vi "Event Handler.vi"(0 "Monkey in":refnum<class "Monkey.lvclass">, 5 "Event type":T1=enum."Message", 7 "Item Name":string, 9 "Data":variant, 11 "error in (no error)":errorcluster) -> (4 "Monkey out":refnum<class "Monkey.lvclass">, 15 "error out":errorcluster)   [LabVIEW 2020, in "Monkey.lvlib" / "Monkey.lvclass"]
doc: "This VI is the event handler of the uService: every time an event is triggered to the uService, this VI is called.\nNote: here you can access the Actor/Class data, but it will be the one coming out from Init. You cannot modify the values.\nThree different events are supported:\nI) Button Pressed: get called on a GUI button pressed. Item Name is the name (label) of the button, Data is empty.\nII) Shared Variable Updated: get called when a SV you subscribed to is updated. Item Name is the name of the SV, and Data is the value (note: you need to convert it to the proper type).\nIII) Message: get called every time a user event is generated using Send Message to Event Handler. The values of Item Name and Data are the one given to the Send Message to Event Handler.\nIV) Ready to launch?: this frame get called every time a new Run is initiated. Each uService is responsible of performing a self check before giving back the green light for the Run to start."
uses:
  Monkey.lvclass
  TALOS/TALOS_PPL.lvlibp/Father of all uServices/Father of all uServices/Event Handler Items.ctl
  Monkey Consumer Case Selector.ctl
  Run Utilities/TypeDefs/Messages/Schedule Message.ctl
  Run Utilities/TypeDefs/DAQ Control.ctl
  Run Utilities/Schedule/Schedule.lvclass
  Run Utilities/TypeDefs/Script Checker Result.ctl
  Inner stop message.ctl
  Run Utilities/Run Block/Run Block.lvclass
  TALOS/TALOS_PPL.lvlibp/Father of all uServices/Father of all uServices/Father of all uServices.lvclass
  Monkey.lvclass/Monkey.ctl
  Run Utilities/Run Utilities.lvlib
  TALOS/TALOS_PPL.lvlibp
  C:/LabVIEW Code/CIRCUS/TALOS/TALOS_PPL.lvlibp/Father of all uServices/Father of all uServices/Father of all uServices.lvclass
  C:/LabVIEW Code/CIRCUS/TALOS/TALOS_PPL.lvlibp/Ancestor/Ancestor/Ancestor.lvclass
  C:/LabVIEW Code/CIRCUS/TALOS/Actor Framework.lvlibp/1abvi3w/vi.lib/ActorFramework/Actor/Actor.lvclass
  C:/LabVIEW Code/CIRCUS/CIRCUS uServices et al/Monkey/Monkey.lvclass
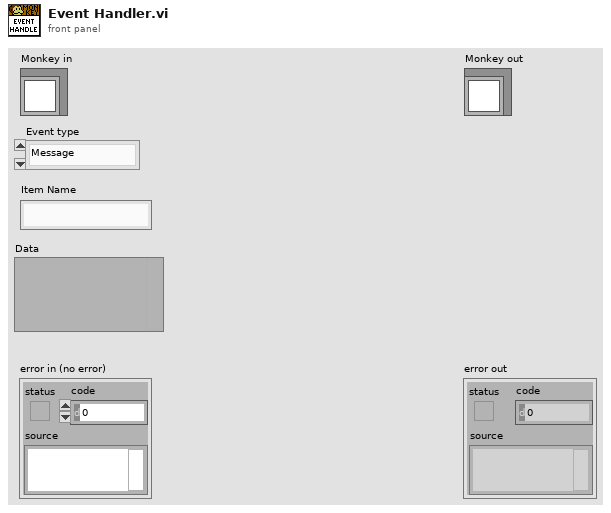
[diagram p1: front panel]
types:
  T1 = typedef "TALOS_PPL.lvlibp/Father of all uServices.lvlib/Father of all uServices.lvclass/Event Handler Items.ctl" = enum16{"Button Pressed", "Message", "Ready to launch?", "Safe Mode", "Start RUN", "Stop RUN"}
  T2 = typedef "Monkey.lvlib/Monkey.lvclass/Monkey Consumer Case Selector.ctl" = enum16{"Init", "Update GUI", "New schedule", "Check Script", "Submit Script", "Banana arrived", "Optimiser - evaluate RUN", "Optimiser - update RUN", "Quality Check", "What to do next", "Update Crit Lvl", "Skip Run", "Stop Schedule", "Skip schedule", "Append"}
  T3 = typedef "Run Utilities.lvlib/Schedule Message.ctl" = cluster{"uS Name":string, "Synchronised":bool, "DAQ Control":T4, "Schedule":refnum<class "Schedule.lvclass">, "Append to top?":bool}
  T4 = typedef "Run Utilities.lvlib/DAQ Control.ctl" = enum16{"On", "Off", "External"}
  T5 = typedef "Run Utilities.lvlib/Script Checker Result.ctl" = enum16{"Passed", "Failed", "Empty"}
  T6 = typedef "Monkey.lvlib/Monkey.lvclass/Inner stop message.ctl" = cluster{"Old value":bool, "Gracefully?":bool}
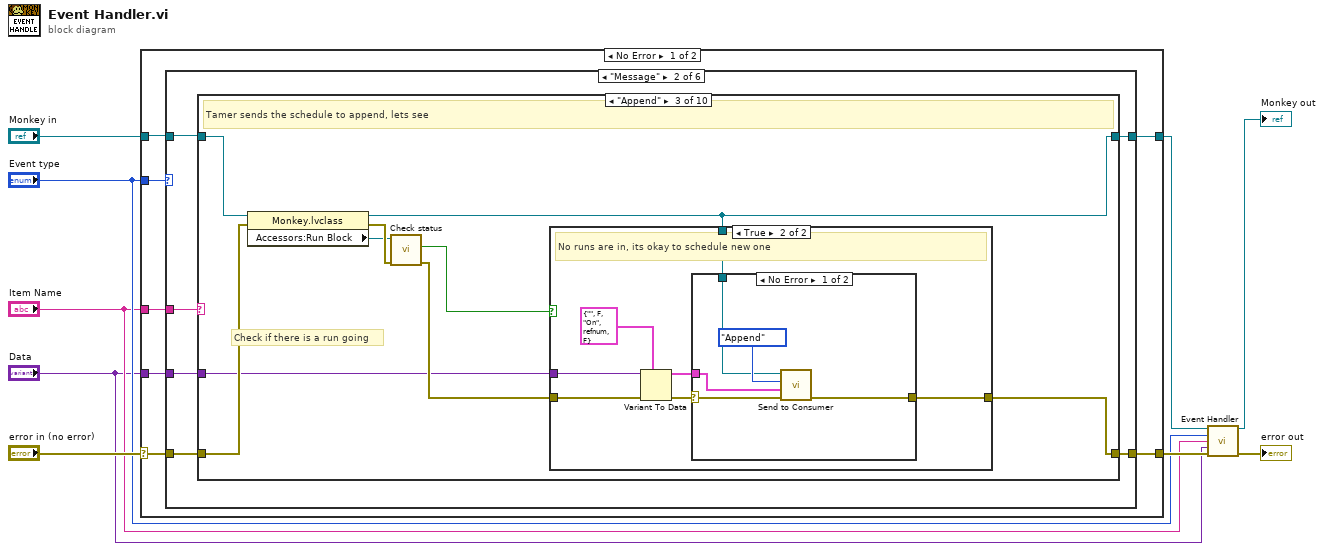
[diagram p0: block diagram]
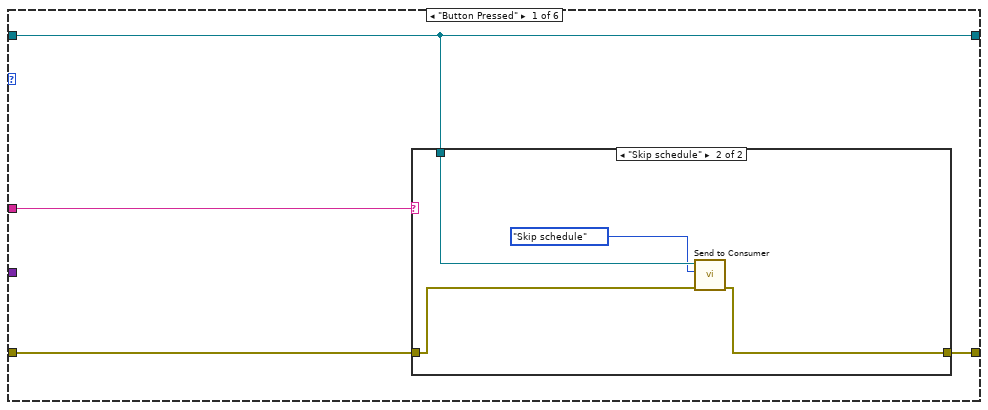
[diagram p2: hidden frame]
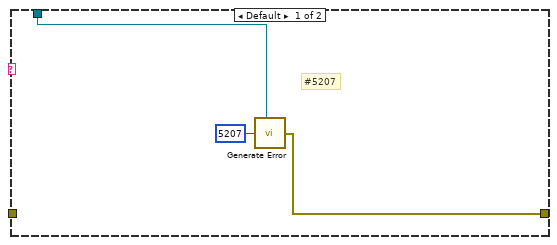
[diagram p3: hidden frame]
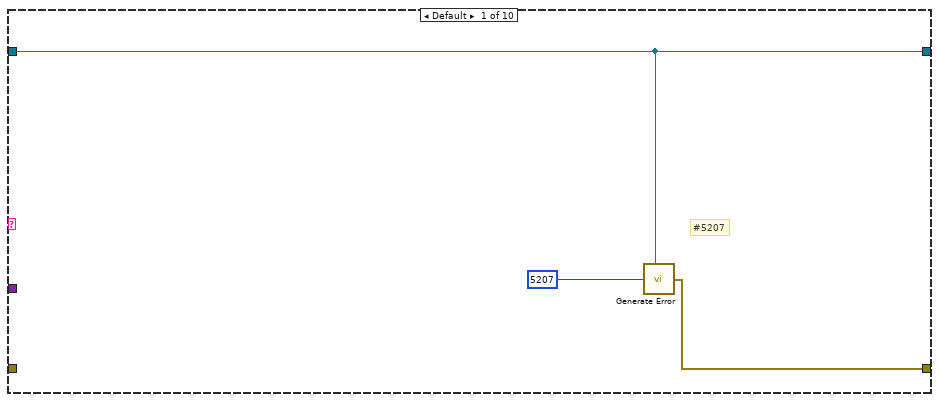
[diagram p4: hidden frame]
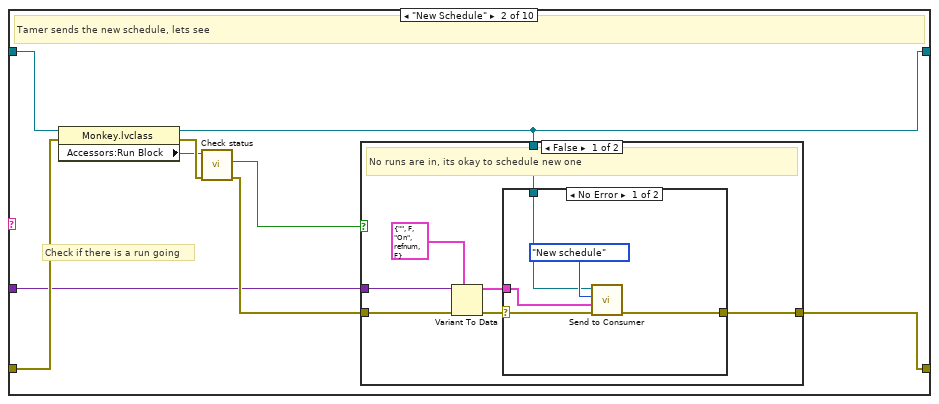
[diagram p5: hidden frame]
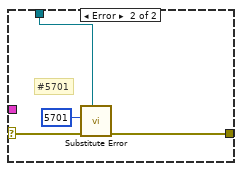
[diagram p6: hidden frame]
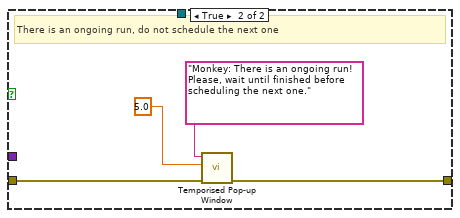
[diagram p7: hidden frame]
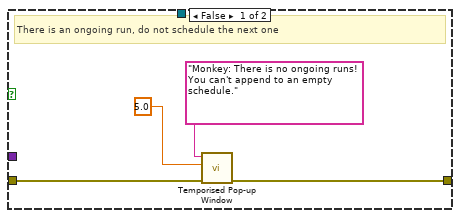
[diagram p8: hidden frame]
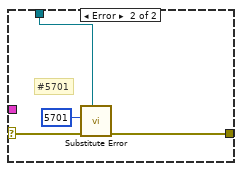
[diagram p9: hidden frame]
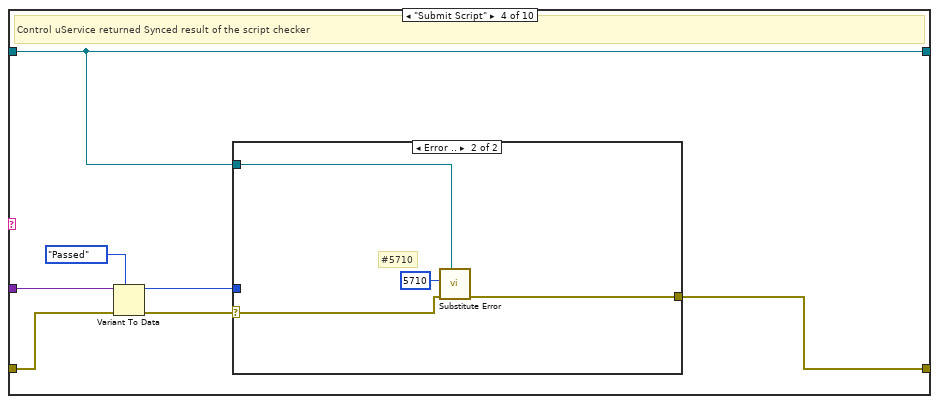
[diagram p10: hidden frame]
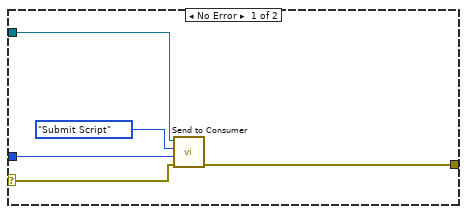
[diagram p11: hidden frame]
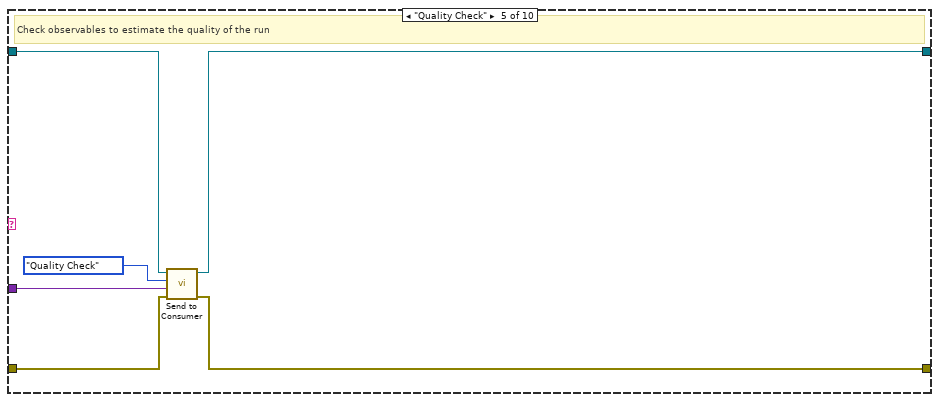
[diagram p12: hidden frame]
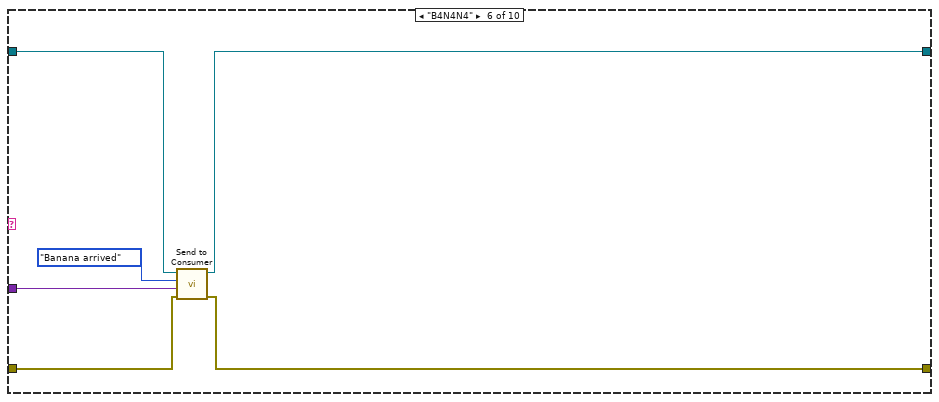
[diagram p13: hidden frame]
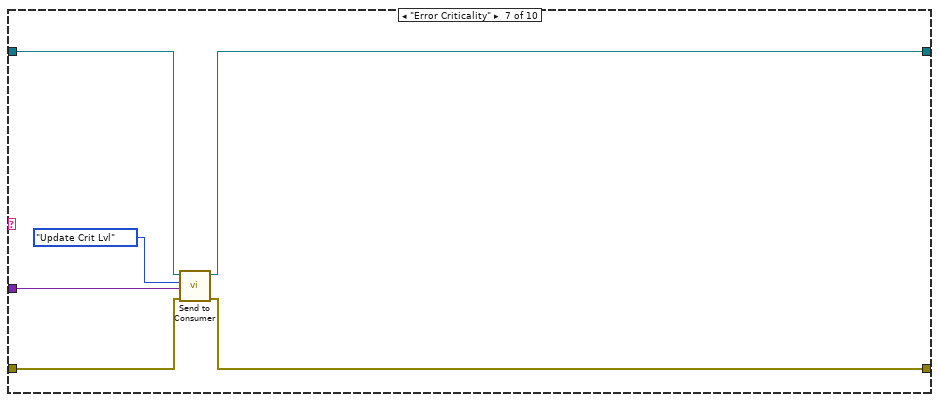
[diagram p14: hidden frame]
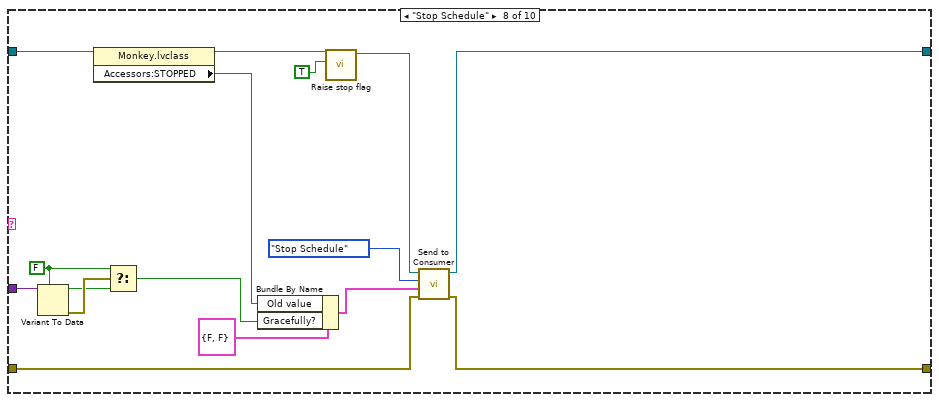
[diagram p15: hidden frame]
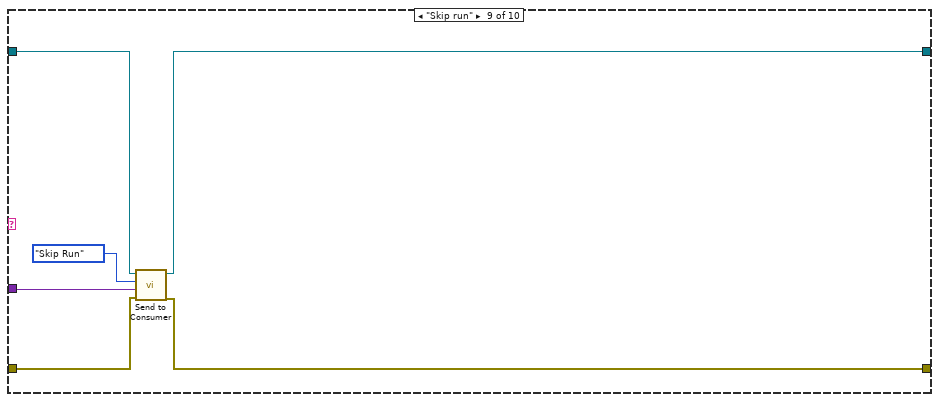
[diagram p16: hidden frame]
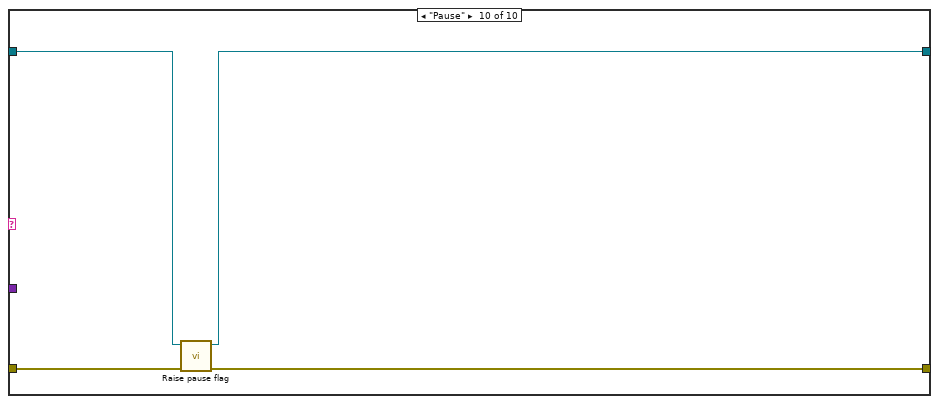
[diagram p17: hidden frame]
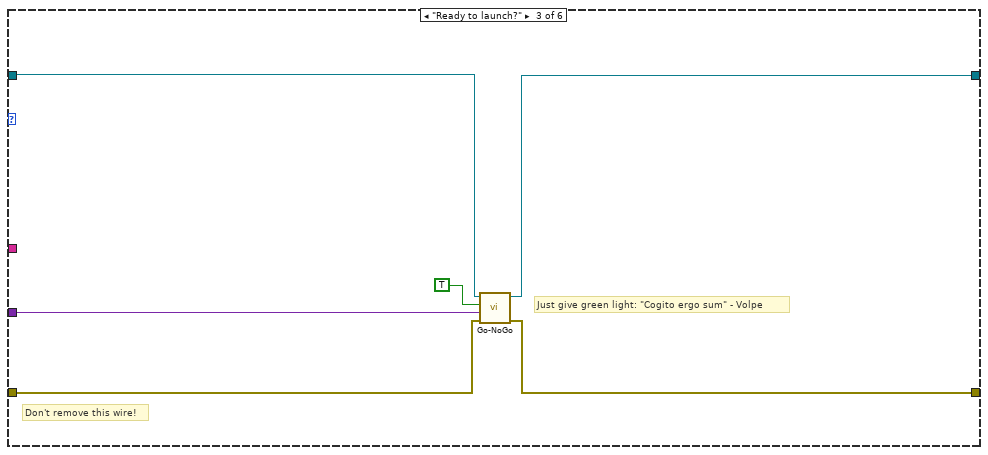
[diagram p18: hidden frame]
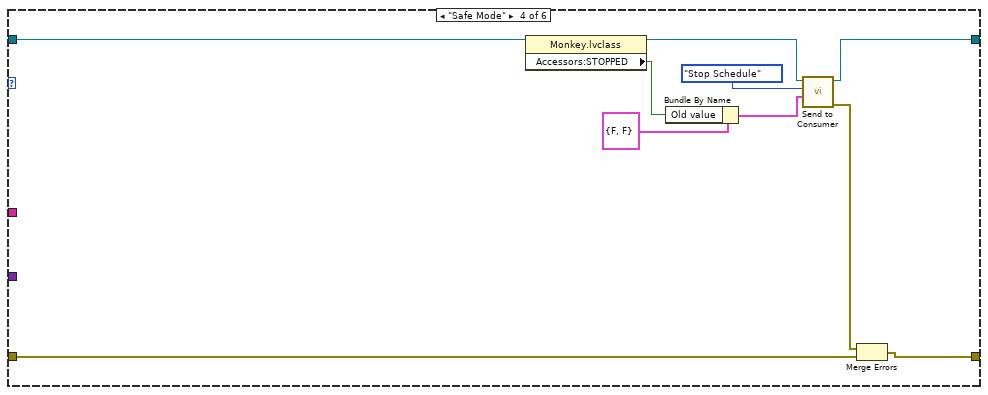
[diagram p19: hidden frame]
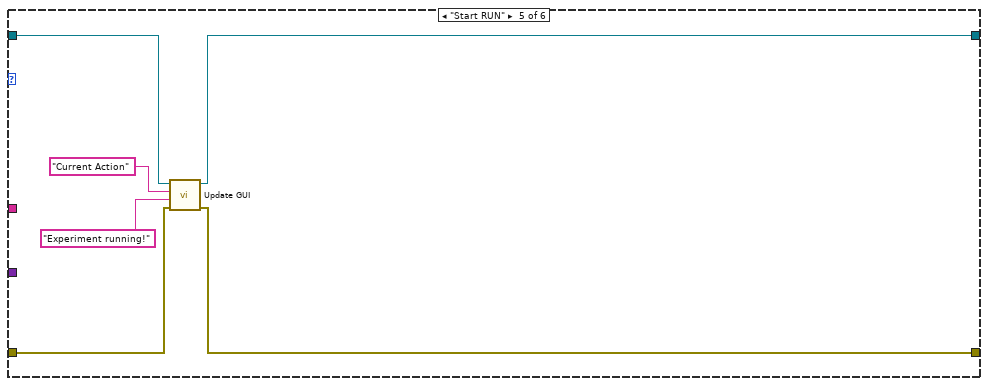
[diagram p20: hidden frame]
diagram:
  n1 = case shown="No Error" "error in (no error)" {
    selector: "error in (no error)" -> [w14 w184]
    tunnel: [w15 w184] -> w7
    tunnel: [w11 w183] -> w4
    tunnel: "Monkey in" -> [w10 w183]
    tunnel: "Event type" -> [w16 _]
    tunnel: "Item Name" -> [w13 _]
    tunnel: "Data" -> [w12 _]
    frame No Error {
      n2 = case shown="\"Message\"" w16 {
        tunnel: [w20 w29 w159 w168 w172 w179] -> w15
        tunnel: w14 -> [w18 w33 w160 w170 w175 w182]
        tunnel: w13 -> [w19 w32 _ _ _ _]
        tunnel: w10 -> [w17 w30 w158 w164 w176 w178]
        tunnel: w12 -> [_ w31 w156 _ _ _]
        tunnel: [w17 w28 w155 w166 w171 w177] -> w11
        frame "Button Pressed" {
          n3 = case shown="\"Skip schedule\"" w19 {
            tunnel: w18 -> [_ w26]
            tunnel: [w21 w25] -> w20
            tunnel: w17 -> [w22 w27]
            frame Default {
              # "#5207"
              n4 = call "Generate Error.vi"("Class"=w22, "Error Code"=5207) -> ("error out"=w21:errorcluster)  [unwired: 5 in]
            }
            frame "Skip schedule" {
              n5 = call "Send to Consumer.vi"("error in (no error)"=w26, "Case ID"=Monkey_Consumer_Case_Selector."Skip schedule" ("Monkey Consumer Case Selector"), "uService Template in"=w27) -> ("error out"=w25:errorcluster)  [unwired: 7 in, 1 out]
            }
          }
        }
        frame "Message" {
          n6 = case shown="\"Append\"" w32 {
            tunnel: w33 -> [_ w45 w74 w100 w114 w121 w128 w144 w150 w153]
            tunnel: w31 -> [_ w42 w71 w101 w116 w119 w127 w135 w149 _]
            tunnel: w30 -> [w34 w38 w67 w95 w112 w118 w124 w141 w145 w154]
            tunnel: [w35 w41 w70 w96 w113 w120 w126 w143 w148 w152] -> w29
            tunnel: [w34 w37 w66 w95 w111 w117 w123 w140 w146 w151] -> w28
            frame Default {
              # "#5207"
              n7 = call "Generate Error.vi"("Class"=w34, "Error Code"=5207) -> ("error out"=w35:errorcluster)  [unwired: 5 in]
            }
            frame "New Schedule" {
              # "Check if there is a run going"
              # "Tamer sends the new schedule, lets see"
              n8 = property class="Monkey.lvclass"(reference=w38, error in=w45) -> (reference out=w37:refnum<class "Monkey.lvclass">, error out=w43:errorcluster, "Accessors:Run Block"=w40:refnum<class "Run Block.lvclass">)
              n9 = call-dynamic "Check status.vi"("error in (no error)"=w43, "Run Block in"=w40) -> ("error out"=w44:errorcluster, "Running"=w39:bool)  [unwired: 7 in, 1 out]
              n10 = case shown="False" w39 {
                tunnel: w42 -> [w52 _]
                tunnel: [w49 w62] -> w41
                tunnel: w37 -> [w48 _]
                tunnel: w44 -> [w47 w65]
                frame False {
                  # "No runs are in, its okay to schedule new one"
                  n11 = Variant To Data(error in=w47, type=T3 {"uS Name"="", "Synchronised"=FALSE, "DAQ Control"=enum."On", "Schedule"=refnum, "Append to top?"=FALSE} ("Monkey Schedule Message"), Variant=w52) -> (data=w50:T3, error out=w51:errorcluster)
                  n12 = case shown="No Error" w51 {
                    selector: w51 -> [w55 w61]
                    tunnel: w50 -> [w54 _]
                    tunnel: w48 -> [w56 w58]
                    tunnel: [w53 w59] -> w49
                    frame No Error {
                      n13 = call "Send to Consumer.vi"("error in (no error)"=w55, "Data"=w54, "Case ID"=Monkey_Consumer_Case_Selector."New schedule" ("Monkey Consumer Case Selector"), "uService Template in"=w56) -> ("error out"=w53:errorcluster)  [unwired: 6 in, 1 out]
                    }
                    frame Error {
                      # "#5701"
                      n14 = call "Substitute Error.vi"("LabVIEW Object"=w58, "error in (no error)"=w61, "Error Code"=5701) -> ("error out"=w59:errorcluster)  [unwired: 8 in]
                    }
                  }
                }
                frame True {
                  # "There is an ongoing run, do not schedule the next one"
                  n15 = call "Temporised Pop-up Window.vi"("error in (no error)"=w65, "Timeout"=5.0, "Text"="Monkey: There is an ongoing run! Please, wait until finished before scheduling the next one.") -> ("error out"=w62:errorcluster)  [unwired: 8 in]
                }
              }
            }
            frame "Append" {
              # "Check if there is a run going"
              # "Tamer sends the schedule to append, lets see"
              n16 = property class="Monkey.lvclass"(reference=w67, error in=w74) -> (reference out=w66:refnum<class "Monkey.lvclass">, error out=w72:errorcluster, "Accessors:Run Block"=w69:refnum<class "Run Block.lvclass">)
              n17 = call-dynamic "Check status.vi"("error in (no error)"=w72, "Run Block in"=w69) -> ("error out"=w73:errorcluster, "Running"=w68:bool)  [unwired: 7 in, 1 out]
              n18 = case shown="True" w68 {
                tunnel: w71 -> [_ w85]
                tunnel: [w75 w82] -> w70
                tunnel: w66 -> [_ w81]
                tunnel: w73 -> [w78 w80]
                frame False {
                  # "There is an ongoing run, do not schedule the next one"
                  n19 = call "Temporised Pop-up Window.vi"("error in (no error)"=w78, "Timeout"=5.0, "Text"="Monkey: There is no ongoing runs! You can't append to an empty schedule.") -> ("error out"=w75:errorcluster)  [unwired: 8 in]
                }
                frame True {
                  # "No runs are in, its okay to schedule new one"
                  n20 = Variant To Data(error in=w80, type=T3 {"uS Name"="", "Synchronised"=FALSE, "DAQ Control"=enum."On", "Schedule"=refnum, "Append to top?"=FALSE} ("Monkey Schedule Message"), Variant=w85) -> (data=w83:T3, error out=w84:errorcluster)
                  n21 = case shown="No Error" w84 {
                    selector: w84 -> [w88 w94]
                    tunnel: w83 -> [w87 _]
                    tunnel: w81 -> [w89 w91]
                    tunnel: [w86 w92] -> w82
                    frame No Error {
                      n22 = call "Send to Consumer.vi"("error in (no error)"=w88, "Data"=w87, "Case ID"=Monkey_Consumer_Case_Selector."Append" ("Monkey Consumer Case Selector"), "uService Template in"=w89) -> ("error out"=w86:errorcluster)  [unwired: 6 in, 1 out]
                    }
                    frame Error {
                      # "#5701"
                      n23 = call "Substitute Error.vi"("LabVIEW Object"=w91, "error in (no error)"=w94, "Error Code"=5701) -> ("error out"=w92:errorcluster)  [unwired: 8 in]
                    }
                  }
                }
              }
            }
            frame "Submit Script" {
              # "Control uService returned Synced result of the script checker"
              n24 = Variant To Data(error in=w100, type=Script_Checker_Result."Passed" ("Script Checker Result"), Variant=w101) -> (data=w97:T5, error out=w98:errorcluster)
              n25 = case shown="Error .." w98 {
                selector: w98 -> [w103 w108]
                tunnel: w97 -> [w105 _]
                tunnel: w95 -> [w104 w109]
                tunnel: [w102 w110] -> w96
                frame No Error {
                  n26 = call "Send to Consumer.vi"("error in (no error)"=w103, "Data"=w105, "Case ID"=Monkey_Consumer_Case_Selector."Submit Script" ("Monkey Consumer Case Selector"), "uService Template in"=w104) -> ("error out"=w102:errorcluster)  [unwired: 6 in, 1 out]
                }
                frame Error {
                  # "#5710"
                  n27 = call "Substitute Error.vi"("LabVIEW Object"=w109, "error in (no error)"=w108, "Error Code"=5710) -> ("error out"=w110:errorcluster)  [unwired: 8 in]
                }
              }
            }
            frame "Quality Check" {
              # "Check observables to estimate the quality of the run"
              n28 = call "Send to Consumer.vi"("error in (no error)"=w114, "Data"=w116, "Case ID"=Monkey_Consumer_Case_Selector."Quality Check" ("Monkey Consumer Case Selector"), "uService Template in"=w112) -> ("error out"=w113:errorcluster, "uService Template out"=w111:refnum<class "Monkey.lvclass">)  [unwired: 6 in]
            }
            frame "B4N4N4" {
              n29 = call "Send to Consumer.vi"("error in (no error)"=w121, "Data"=w119, "Case ID"=Monkey_Consumer_Case_Selector."Banana arrived" ("Monkey Consumer Case Selector"), "uService Template in"=w118) -> ("error out"=w120:errorcluster, "uService Template out"=w117:refnum<class "Monkey.lvclass">)  [unwired: 6 in]
            }
            frame "Error Criticality" {
              n30 = call "Send to Consumer.vi"("error in (no error)"=w128, "Data"=w127, "Case ID"=Monkey_Consumer_Case_Selector."Update Crit Lvl" ("Monkey Consumer Case Selector"), "uService Template in"=w124) -> ("error out"=w126:errorcluster, "uService Template out"=w123:refnum<class "Monkey.lvclass">)  [unwired: 6 in]
            }
            frame "Stop Schedule" {
              w136 = FALSE
              n31 = Variant To Data(type=w136, Variant=w135) -> (data=w137:bool, error out=w138:errorcluster)  [unwired: 1 in]
              n32 = property class="Monkey.lvclass"(reference=w141) -> (reference out=w131:refnum<class "Monkey.lvclass">, "Accessors:STOPPED"=w133:bool)  [unwired: 1 in, 1 out]
              n33 = Select(t=w136, s=w138, f=w137) -> (s? t:f=w134:bool)
              n34 = Bundle By Name(cluster=T6 {"Old value"=FALSE, "Gracefully?"=FALSE} ("Stop msg"), "Old value"=w133, "Gracefully?"=w134) -> (w132:T6)
              n35 = call-dynamic "Raise stop flag.vi"("on/off"=TRUE, "Monkey in"=w131) -> ("Monkey out"=w130:refnum<class "Monkey.lvclass">)  [unwired: 8 in, 1 out]
              n36 = call "Send to Consumer.vi"("error in (no error)"=w144, "Data"=w132, "Case ID"=Monkey_Consumer_Case_Selector."Stop Schedule" ("Monkey Consumer Case Selector"), "uService Template in"=w130) -> ("error out"=w143:errorcluster, "uService Template out"=w140:refnum<class "Monkey.lvclass">)  [unwired: 6 in]
            }
            frame "Skip run" {
              n37 = call "Send to Consumer.vi"("error in (no error)"=w150, "Data"=w149, "Case ID"=Monkey_Consumer_Case_Selector."Skip Run" ("Monkey Consumer Case Selector"), "uService Template in"=w145) -> ("error out"=w148:errorcluster, "uService Template out"=w146:refnum<class "Monkey.lvclass">)  [unwired: 6 in]
            }
            frame "Pause" {
              n38 = call-dynamic "Raise pause flag.vi"("error in (no error)"=w153, "Monkey in"=w154) -> ("error out"=w152:errorcluster, "Monkey out"=w151:refnum<class "Monkey.lvclass">)  [unwired: 8 in]
            }
          }
        }
        frame "Ready to launch?" {
          # "Don't remove this wire!"
          # "Just give green light: \"Cogito ergo sum\" - Volpe"
          n39 = call-dynamic "Go-NoGo.vi"("error in (no error)"=w160, "Go-NoGo Data"=w156, "Go?"=TRUE, "Father of all uServices in"=w158) -> ("error out"=w159:errorcluster, "Father of all uServices out"=w155:refnum<class "Monkey.lvclass">)  [unwired: 6 in]
        }
        frame "Safe Mode" {
          n40 = property class="Monkey.lvclass"(reference=w164) -> (reference out=w163:refnum<class "Monkey.lvclass">, "Accessors:STOPPED"=w162:bool)  [unwired: 1 in, 1 out]
          n41 = Bundle By Name(cluster=T6 {"Old value"=FALSE, "Gracefully?"=FALSE} ("Stop msg"), "Old value"=w162) -> (w161:T6)
          n42 = call "Send to Consumer.vi"("Data"=w161, "Case ID"=Monkey_Consumer_Case_Selector."Stop Schedule" ("Monkey Consumer Case Selector"), "uService Template in"=w163) -> ("error out"=w167:errorcluster, "uService Template out"=w166:refnum<class "Monkey.lvclass">)  [unwired: 7 in]
          n43 = Merge Errors(w167, w170) -> (w168:errorcluster)
        }
        frame "Start RUN" {
          n44 = call "Update GUI.vi"("error in (no error)"=w175, "Data"="Experiment running!" ("GUI Item Name"), "GUI Item Name"="Current Action", "uService Template in"=w176) -> ("error out"=w172:errorcluster, "uService Template out"=w171:refnum<class "Monkey.lvclass">)  [unwired: 6 in]
        }
        frame "Stop RUN" {
          n45 = call "Update GUI.vi"("error in (no error)"=w182, "Data"="Experiment finished! Ending the script..." ("GUI Item Name"), "GUI Item Name"="Current Action", "uService Template in"=w178) -> ("error out"=w179:errorcluster, "uService Template out"=w177:refnum<class "Monkey.lvclass">)  [unwired: 6 in]
        }
      }
    }
    frame Error {
    }
  }
  n46 = call-parent "Event Handler.vi"("uService Template in"=w4, "Event type"="Event type", "Item Name"="Item Name", "Data"="Data", "error in (no error)"=w7) -> ("uService Template out"=→"Monkey out":refnum<class "Monkey.lvclass">, "error out"=→"error out":errorcluster)  [unwired: 9 in]
